vi "sequence_struct_demo.vi"() -> ()   [LabVIEW 2013]
panel:
  out "czas[ms]":u32
  out "wynik":dbl
  out "przejscie petli":dbl
  in  "ilosc wykonan":dbl
  in  "zakres do":dbl
  in  "zakres od":dbl
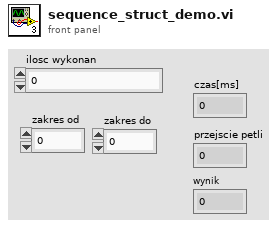
[diagram p1: front panel]
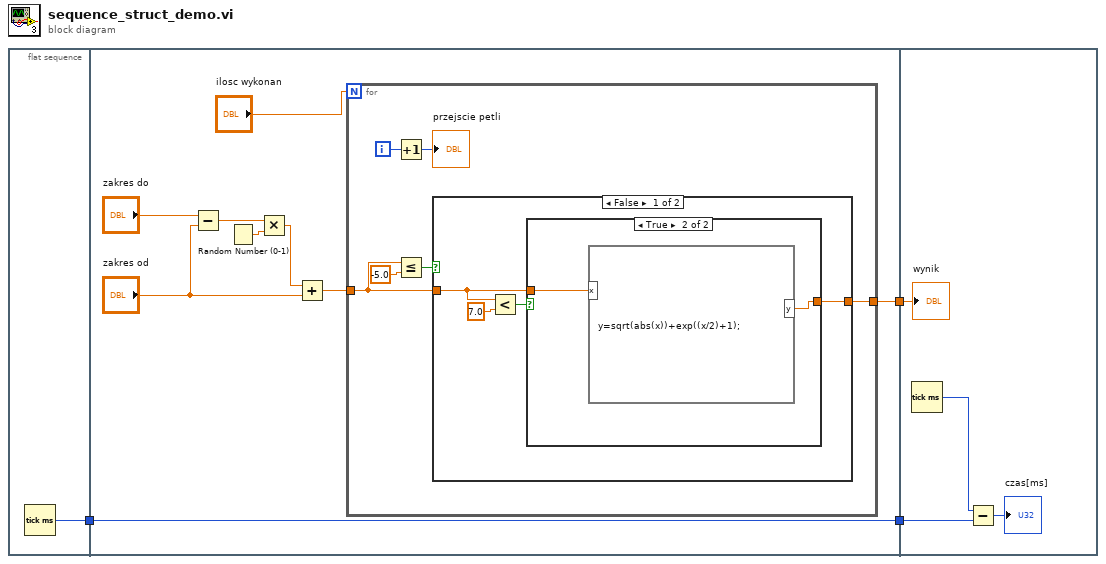
[diagram p0: block diagram]
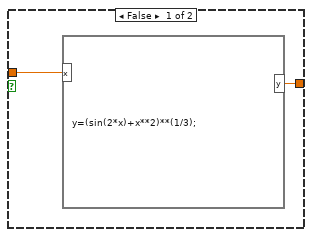
[diagram p2: hidden frame]
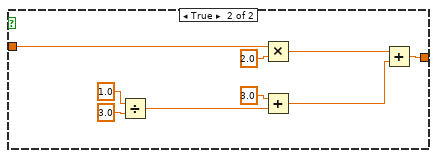
[diagram p3: hidden frame]
diagram:
  n1 = flat-sequence {
    tunnel: [w4] -> w1
    tunnel: [w13] -> w3
    tunnel: [w7] -> w2
    tunnel: w1 -> [w7]
    tunnel: w3 -> [w40]
    tunnel: w2 -> [w37]
    frame #0 {
      n2 = Tick Count (ms)() -> (millisecond timer value=w4:u32)
    }
    frame #1 {
      n3 = Subtract(x="zakres do", y="zakres od") -> (x-y=w10:dbl)
      n4 = Random Number (0-1)() -> (number: 0 to 1=w11:dbl)
      n5 = Multiply(x=w10, y=w11) -> (x*y=w12:dbl)
      n6 = Add(x=w12, y="zakres od") -> (x+y=w6:dbl)
      n7 = for {
        N: "ilosc wykonan" -> [_]
        tunnel: [w19] -> w13
        tunnel: w6 -> [w16]
        i -> [w15]
        n8 = Increment(x=w15) -> (x+1=→"przejscie petli":i32)
        n9 = Less Or Equal?(x=w16, y=-5.0) -> (x <= y?=w18:bool)
        n10 = case shown="False" w18 {
          tunnel: w16 -> [w21 w36]
          tunnel: [w20 w28] -> w19
          frame False {
            n11 = Less?(x=w21, y=7.0) -> (x < y?=w23:bool)
            n12 = case shown="True" w23 {
              tunnel: w21 -> [w25 w27]
              tunnel: [w24 w26] -> w20
              frame False {
                n13 = formula code="y=(sin(2*x)+x**2)**(1/3);"("x"=w25) -> ("y"=w24:dbl)
              }
              frame True {
                n14 = formula code="y=sqrt(abs(x))+exp((x/2)+1);"("x"=w27) -> ("y"=w26:dbl)
              }
            }
          }
          frame True {
            n15 = Divide(x=1.0 ("y"), y=3.0) -> (x/y=w29:dbl)
            n16 = Multiply(x=w36, y=2.0) -> (x*y=w34:dbl)
            n17 = Add(x=3.0 ("y"), y=w29) -> (x+y=w32:dbl)
            n18 = Add(x=w34, y=w32) -> (x+y=w28:dbl)
          }
        }
      }
    }
    frame #2 {
      n19 = Tick Count (ms)() -> (millisecond timer value=w38:u32)
      n20 = Subtract(x=w38, y=w37) -> (x-y=→"czas[ms]":u32)
      "wynik" <- w40
    }
  }
